vi "SetCrcType.vi"(8 "error in (no error)":errorcluster, 11 "reference in":refnum<class "VdMultiMeter.lvclass">) -> (0 "error out":errorcluster, 3 "reference out":refnum<class "VdMultiMeter.lvclass">)   [LabVIEW 2020, in "MulitMeters.lvlib" / "VdMultiMeter.lvclass"]
uses:
  VdMultiMeter.lvclass
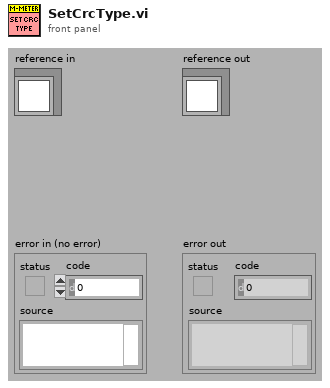
[diagram p1: front panel]
types:
  T1 = typedef "MulitMeters.lvlib/VdMultiMeter.lvclass/ObjectAttributes.ctl" = cluster{"ChecksumCalculationType":refnum<class "ChecksumCalculation.lvclass">}
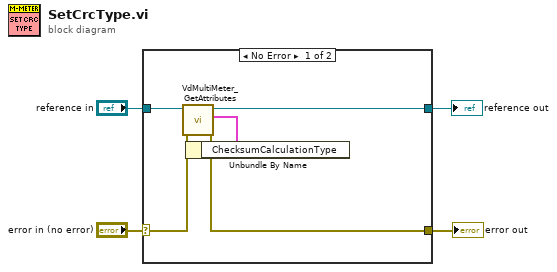
[diagram p0: block diagram]
diagram:
  n1 = case shown="No Error" "error in (no error)" {
    selector: "error in (no error)" -> [w9 w11]
    tunnel: [w7 w11] -> w3
    tunnel: [w5 w10] -> w1
    tunnel: "reference in" -> [w6 w10]
    frame No Error {
      n2 = call "VdMultiMeter_GetAttributes.vi"("error in (no error)"=w9, "reference in"=w6) -> ("error out"=w7:errorcluster, "Data"=w8:T1, "reference out"=w5:refnum<class "VdMultiMeter.lvclass">)  [unwired: 6 in, 1 out]
      n3 = Unbundle By Name(w8) -> ()  [unwired: 1 out]
    }
    frame Error {
    }
  }
  "error out" <- w3
  "reference out" <- w1
